vi "Data Source Import.vi"(11 "Data In":string[][](array[string])) -> (2 "OK?":bool, 3 "Data":string[][](array[string]))   [LabVIEW 2020]
uses:
  <vilib>/Utility/miscctls.llb/LVRowAndColumnUnsignedTypeDef.ctl
panel:
  in  "Data Source":i32(listbox)
  in  "Import2":bool
  in  "Import":bool
  in  "Cancle":bool
  in  "OK":bool
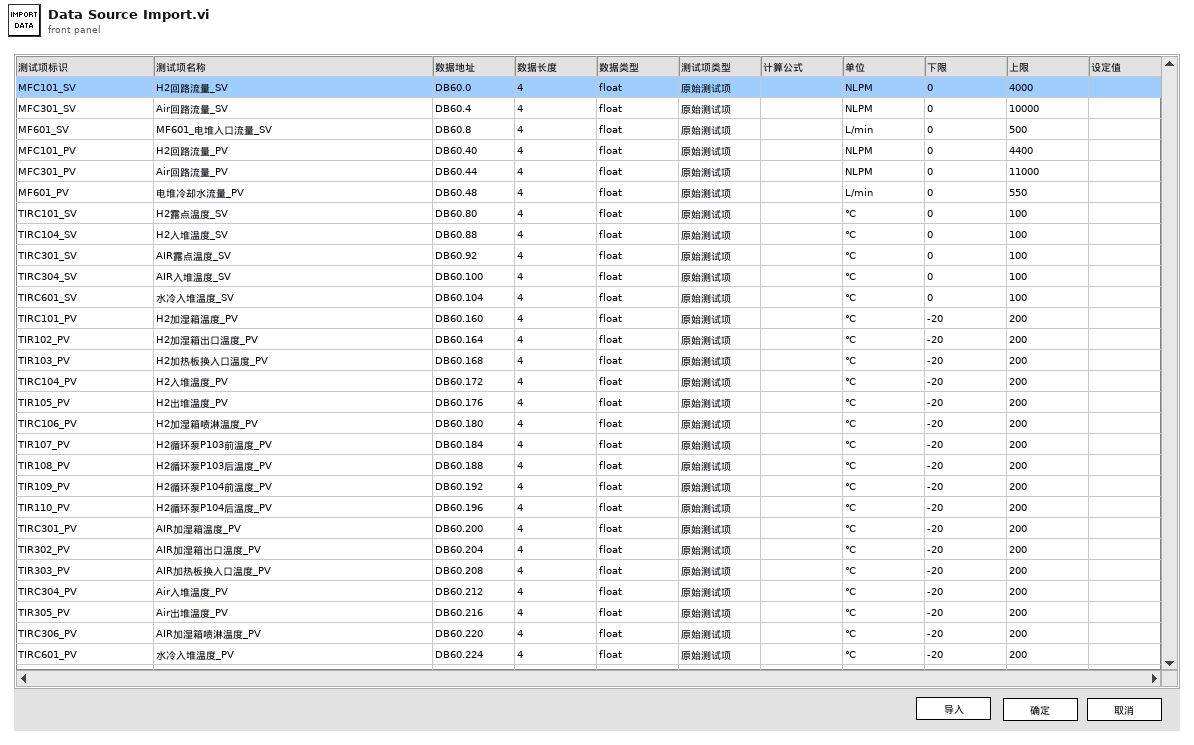
[diagram p1: front panel]
types:
  T1 = typedef "LVRowAndColumnUnsignedTypeDef.ctl" = cluster{"Row":u32, "Column":u32}
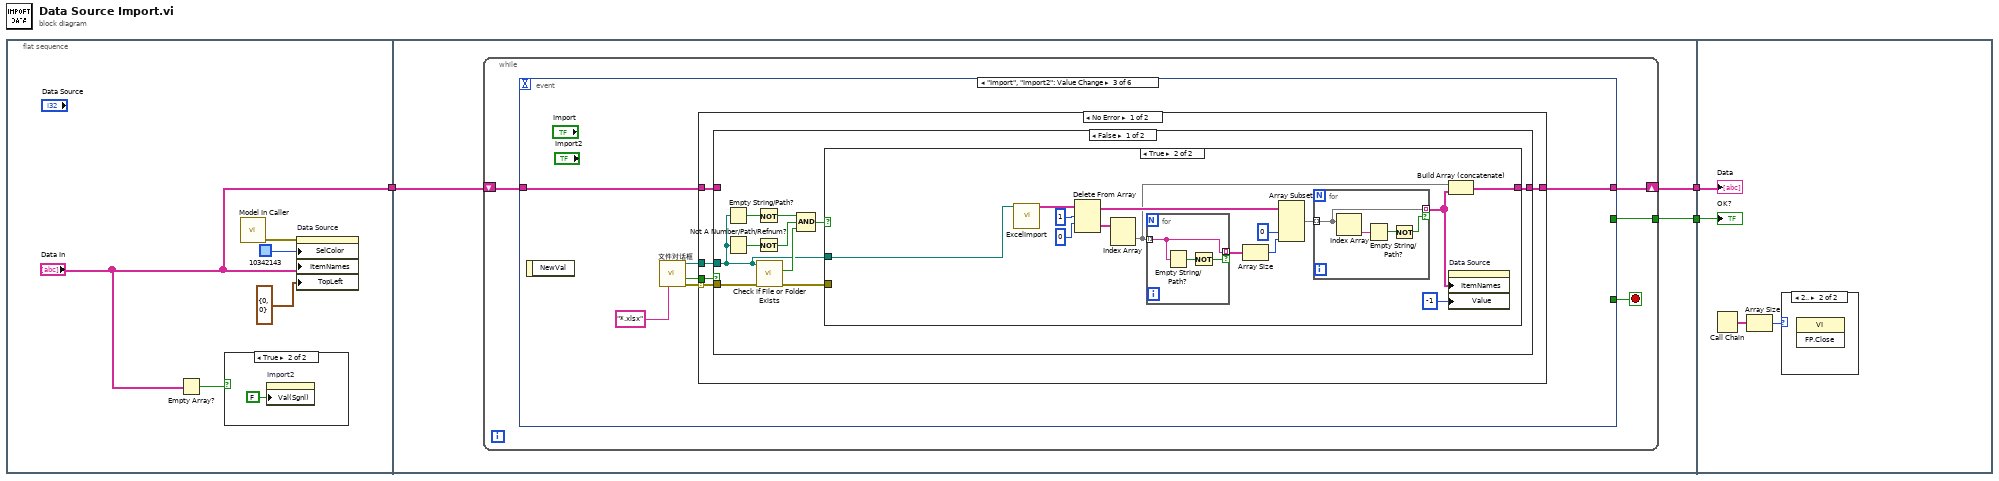
[diagram p0: block diagram]
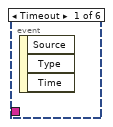
[diagram p3: hidden frame]
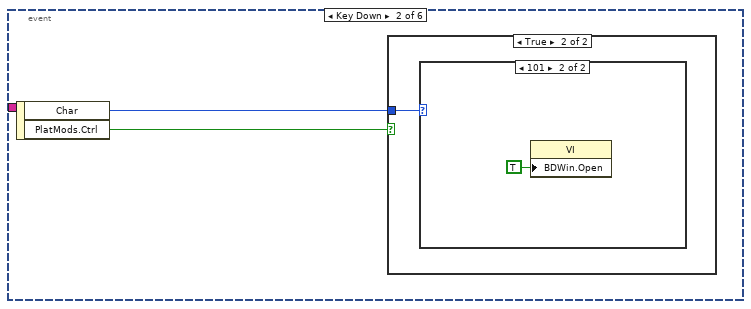
[diagram p4: hidden frame]
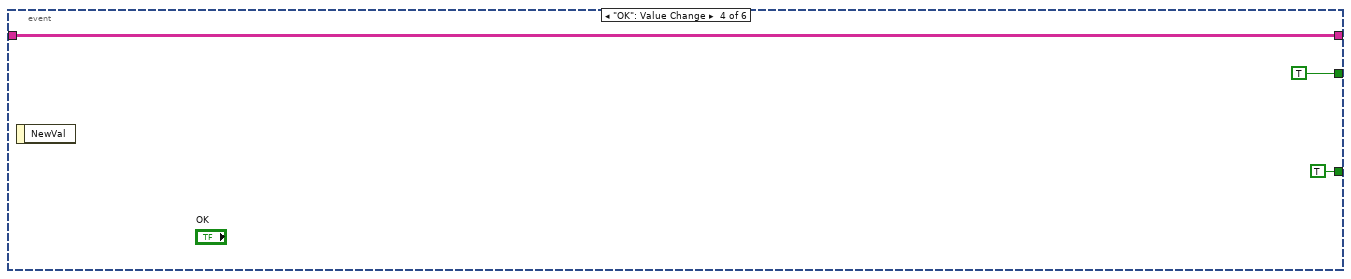
[diagram p10: hidden frame]
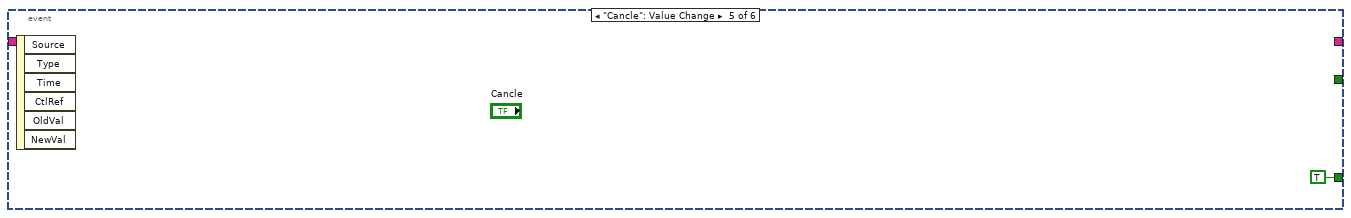
[diagram p11: hidden frame]
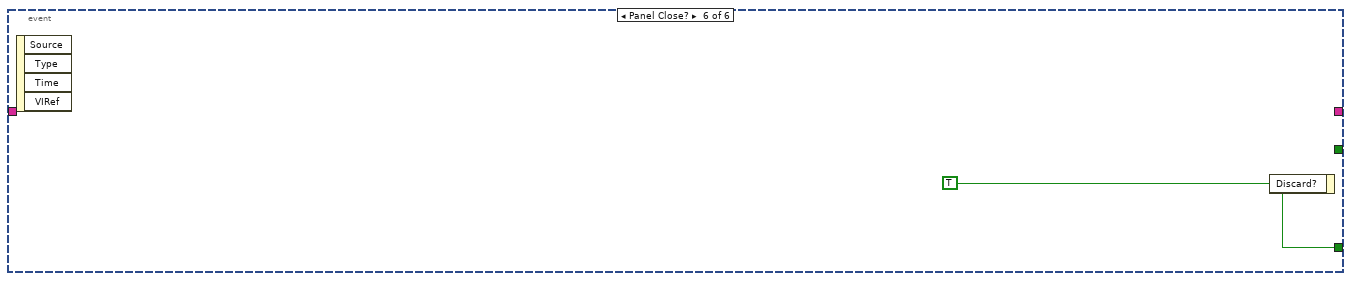
[diagram p12: hidden frame]
diagram:
  n1 = flat-sequence {
    tunnel: ["Data In"] -> w1
    tunnel: [w12] -> w3
    tunnel: [w11] -> w2
    tunnel: w1 -> [w10]
    tunnel: w3 -> [w69]
    tunnel: w2 -> [w68]
    frame #0 {
      n2 = Empty Array?(array="Data In") -> (empty?=w5:bool)
      n3 = case shown="True" w5 {
        frame False {
        }
        frame True {
          n4 = property on="Import2" class="Bool (严格)"("Val(Sgnl)"=FALSE ("值(信号)")) -> ()  [unwired: 2 in, 2 out]
        }
      }
      n5 = call "Model In Caller.vi"() -> ("error out"=w4:errorcluster)  [unwired: 11 in]
      n6 = property on="Data Source" class="MCListbox (严格)"(error in=w4, "SelColor"=u32 10342143 ("选择颜色"), "ItemNames"="Data In", "TopLeft"=T1 {"Row"=0, "Column"=0} ("左上可见单元格")) -> ()  [unwired: 1 in, 2 out]
    }
    frame #1 {
      n7 = while {
        tunnel: [w15] -> w12
        shift-right: [w14] -> w11
        shift-left: w10 -> [w13]
        stop <- w16 stop-if-true
        n8 = event shown="[2] \"Import\", \"Import2\": Value Change" {
          selector: _ -> [_ _ _ _ _ _]
          dyn-events: _ -> [_ _ _ _ _ _]
          timeout: _ -> [_ _ _ _ _ _]
          tunnel: [_ _ _ TRUE ("放弃？") TRUE ("放弃？") w67] -> w16
          tunnel: [_ _ _ TRUE _ _] -> w15
          tunnel: [_ _ w22 w64 _ _] -> w14
          tunnel: w13 -> [_ _ w21 w64 _ _]
          event Timeout {
            n9 = event-data() -> ()  [unwired: 1 in, 3 out]
          }
          event Key Down {
            n10 = event-data() -> ("Char"=w18:i16, "PlatMods.Ctrl"=w17:bool)  [unwired: 1 in]
            n11 = case shown="True" w17 {
              tunnel: w18 -> [_ w19]
              frame False {
              }
              frame True {
                n12 = case shown="101" w19 {
                  frame 0, Default {
                  }
                  frame 101 {
                    n13 = property class="VI"("BDWin.Open"=TRUE ("程序框图窗口:打开")) -> ()  [unwired: 2 in, 2 out]
                  }
                }
              }
            }
          }
          event "Import", "Import2": Value Change {
            n14 = event-data() -> ()  [unwired: 1 in, 1 out]
            n15 = call "文件对话框"("pattern (all files)"="*.xlsx") -> ("selected path"=w26:path, "cancelled"=w24:bool, "error out"=w25:errorcluster)  [unwired: 11 in, 1 out]
            n16 = case shown="No Error" w25 {
              selector: w25 -> [w29 _]
              tunnel: w24 -> [w31 _]
              tunnel: w26 -> [w30 _]
              tunnel: [w28 _] -> w22
              tunnel: w21 -> [w27 _]
              frame No Error {
                n17 = case shown="False" w31 {
                  tunnel: w30 -> [w36 _]
                  tunnel: w29 -> [w34 _]
                  tunnel: [w32 _] -> w28
                  tunnel: w27 -> [_ _]
                  frame False {
                    n18 = Empty String/Path?(string/path=w36) -> (empty?=w41:bool)
                    n19 = Not A Number/Path/Refnum?(number/path/refnum=w36) -> (NaN/Path/Refnum?=w40:bool)
                    n20 = Not(x=w41) -> (.not. x?=w39:bool)
                    n21 = Not(x=w40) -> (.not. x?=w38:bool)
                    n22 = call <vilib>:"Check if File or Folder Exists.vi"("error in (no error)"=w34, "path"=w36) -> ("error out"=w33:errorcluster, "file or folder exists?"=w37:bool)  [unwired: 7 in, 1 out]
                    n23 = Compound Arithmetic op=AND ("复合运算")(w39, w38, w37) -> (w35:bool)
                    n24 = case shown="True" w35 {
                      tunnel: w36 -> [_ w43]
                      tunnel: w33 -> [_ _]
                      tunnel: [_ w44] -> w32
                      frame False {
                      }
                      frame True {
                        n25 = call "ExcelImport.vi"("路径"=w43) -> ("All"=w42:string[][])  [unwired: 7 in, 3 out]
                        n26 = Delete From Array(array=w42, length=1 ("长度"), index (row)=0 ("索引 (行)")) -> (deleted portion=w47:string[][], array with subset deleted=w52:string[][])  [unwired: 1 in]
                        n27 = Index Array(array=w47) -> (element=w45:string[])  [unwired: 2 in]
                        n28 = for {
                          tunnel: [w56] -> w50 mode=indexing if=w57
                          tunnel: w45 -> [w56] mode=indexing
                          n29 = Empty String/Path?(string/path=w56) -> (empty?=w58:bool)
                          n30 = Not(x=w58) -> (.not. x?=w57:bool)
                        }
                        n31 = Array Size(array=w50) -> (size(s)=w49:i32)
                        n32 = Array Subset(array=w52, index (col)=0 ("索引"), length (col)=w49) -> (w48:string[][])  [unwired: 2 in]
                        n33 = for {
                          tunnel: w48 -> [w62] mode=indexing
                          tunnel: [w62] -> w46 mode=indexing if=w59
                          n34 = Index Array(array=w62) -> (element=w61:string)  [unwired: 1 in]
                          n35 = Empty String/Path?(string/path=w61) -> (empty?=w60:bool)
                          n36 = Not(x=w60) -> (.not. x?=w59:bool)
                        }
                        n37 = Build Array (concatenate)(w45, w46) -> (w44:string[][])
                        n38 = property on="Data Source" class="MCListbox (严格)"("ItemNames"=w46, "Value"=-1 ("Data Source")) -> ()  [unwired: 2 in, 2 out]
                      }
                    }
                  }
                  frame True {
                  }
                }
              }
              frame Error {
              }
            }
          }
          event "OK": Value Change {
            n39 = event-data() -> ()  [unwired: 1 in, 1 out]
          }
          event "Cancle": Value Change {
            n40 = event-data() -> ()  [unwired: 1 in, 6 out]
          }
          event Panel Close? {
            w67 = TRUE ("放弃？")
            n41 = event-data() -> ()  [unwired: 1 in, 4 out]
            n42 = event-data("Discard?"=w67) -> ()  [unwired: 1 in, 1 out]
          }
        }
      }
    }
    frame #2 {
      n43 = Call Chain() -> (call chain=w70:string[])
      n44 = Array Size(array=w70) -> (size(s)=w71:i32)
      n45 = case shown="2.." w71 {
        frame 0, Default {
        }
        frame 2.. {
          n46 = invoke class="VI" method="FP.Close"() -> ()  [unwired: 3 in, 3 out]
        }
      }
      "OK?" <- w69
      "Data" <- w68
    }
  }
